vi "Beta Calcul.vi"(11 "Velocity in":cluster{"x":dbl, "y":dbl}={"x"=10.0, "y"=10.0}) -> (2 "Beta out":dbl)   [LabVIEW 2021, in "Game Board.lvclass"]
doc: "MIT Licence\nCopyright (c) 2024 David Grollier"
uses:
  Game Board.lvclass
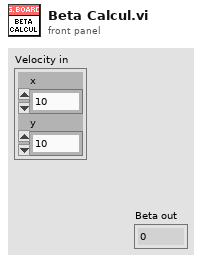
[diagram p1: front panel]
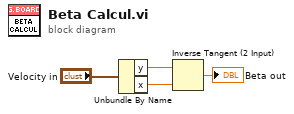
[diagram p0: block diagram]
diagram:
  n1 = Unbundle By Name("Velocity in") -> ("y"=w3:dbl, "x"=w2:dbl)
  n2 = Inverse Tangent (2 Input)(1:w2, 2:w3) -> (0:→"Beta out":dbl)
